vi "Untitled 1.vi"(8 "error in":errorcluster, 11 "fpga reference":refnum<k20>) -> (0 "error out":errorcluster, 2 "Chassis Temperature":sgl)   [LabVIEW 2017, in "DeviceHealth.lvlib"]
uses:
  <vilib>/addons/InsightCM/Devices/Shared/Common/DeviceHealth/DeviceHealth.lvlib
  <vilib>/Utility/error.llb/Error Cluster From Error Code.vi
  <vilib>/rvi/errors/niLvFpgaAdjustHostInterfaceError.vi
  <vilib>/rvi/interface/nirviReadWriteControl/nirviReadWriteControl.xnode
  NiFpgaLv.dll
  <vilib>/rvi/interface/Simulation/niFpgaSimulationCallBeginRW.vi
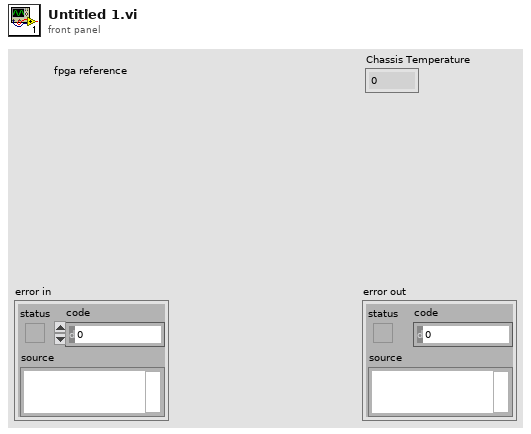
[diagram p1: front panel]
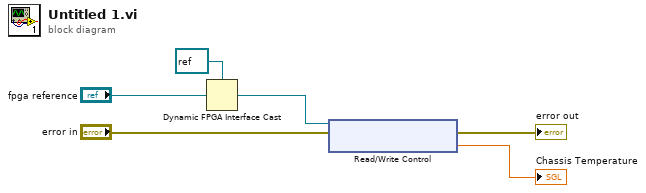
[diagram p0: block diagram]
diagram:
  n1 = Dynamic FPGA Interface Cast(Session In=refnum<k20> refnum ("Type"), Type="fpga reference") -> (Session Out=w4:refnum<k20>)
  n2 = xnode "Read/Write Control"("FPGA VI Reference In"=w4, "error in"="error in") -> ("error out"=→"error out":errorcluster, "Chassis Temperature"=→"Chassis Temperature":sgl)  [unwired: 1 out]
